vi "Zamojski_10_sub_2.vi"(8 "error in (no error)":errorcluster) -> (0 "error out":errorcluster)   [LabVIEW 2020]
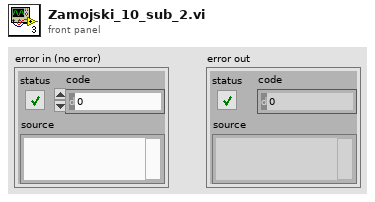
[diagram p1: front panel]
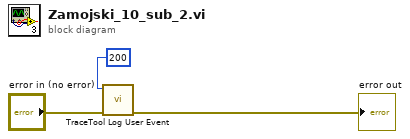
[diagram p0: block diagram]
diagram:
  n1 = call <vilib>:"TraceTool Log User Event.vi"("error in (no error)"="error in (no error)", "Event ID (0-255)"=u32 200) -> ("error out"=→"error out":errorcluster)  [unwired: 9 in]
